vi "Import Configuration RTM.vi"(8 "error in (no error)":errorcluster, 11 "Node Ptr":u64 format="%.0x") -> (0 "error out":errorcluster)   [LabVIEW 2017, in "NI-SWITCH System Explorer.lvlib"]
uses:
  NI-SWITCH System Explorer.lvlib
  Scripting/NI-SWITCH Scripting.lvlib
panel:
  in  "Path":path
  in  "Tag":string
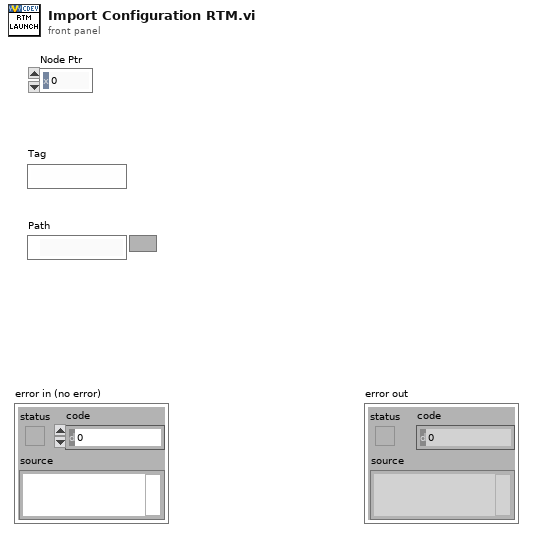
[diagram p1: front panel]
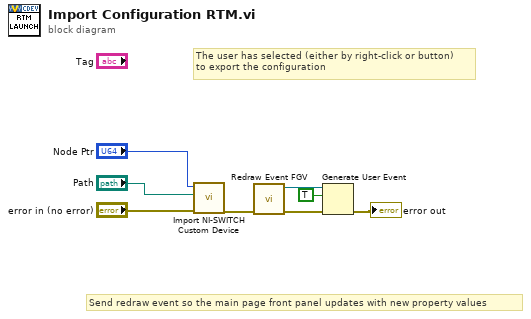
[diagram p0: block diagram]
diagram:
  # "Send redraw event so the main page front panel updates with new property values"
  # "The user has selected (either by right-click or button)\nto export the configuration"
  n1 = call "Import NI-SWITCH Custom Device.vi"("error in"="error in (no error)", "datalog path (use dialog)"="Path", "ni-switch custom device in"="Node Ptr") -> ("error out"=w1:errorcluster)  [unwired: 7 in, 1 out]
  n2 = call "Redraw Event FGV.vi"("error in (no error)"=w1) -> ("error out"=w8:errorcluster, "Redraw Event"=w6:refnum<user-event>)  [unwired: 9 in]
  n3 = Generate User Event(user event=w6, event data cluster=TRUE ("event data"), error in=w8) -> (error out=→"error out":errorcluster)  [unwired: 1 in, 1 out]
